vi "Binned Values.vi"(3 "Tolerance":dbl=1.0 format="%.2f", 4 "Precision (3)":string, 5 "String Array In":string[](array[string])) -> (2 "String Array Out":string[](array[string]))   [LabVIEW 2022 SP3]
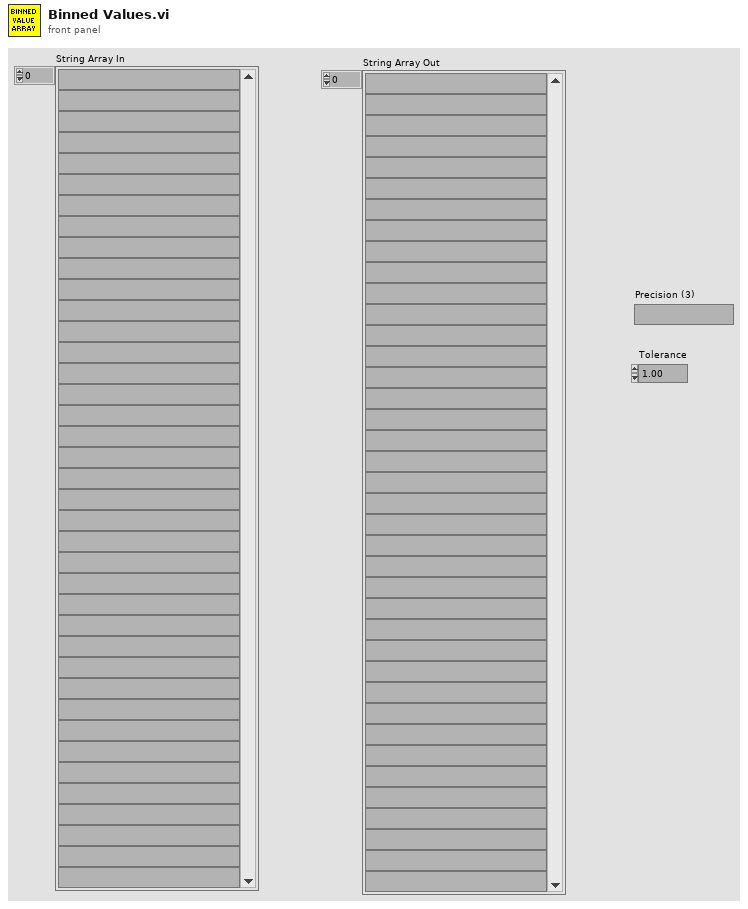
[diagram p1: front panel]
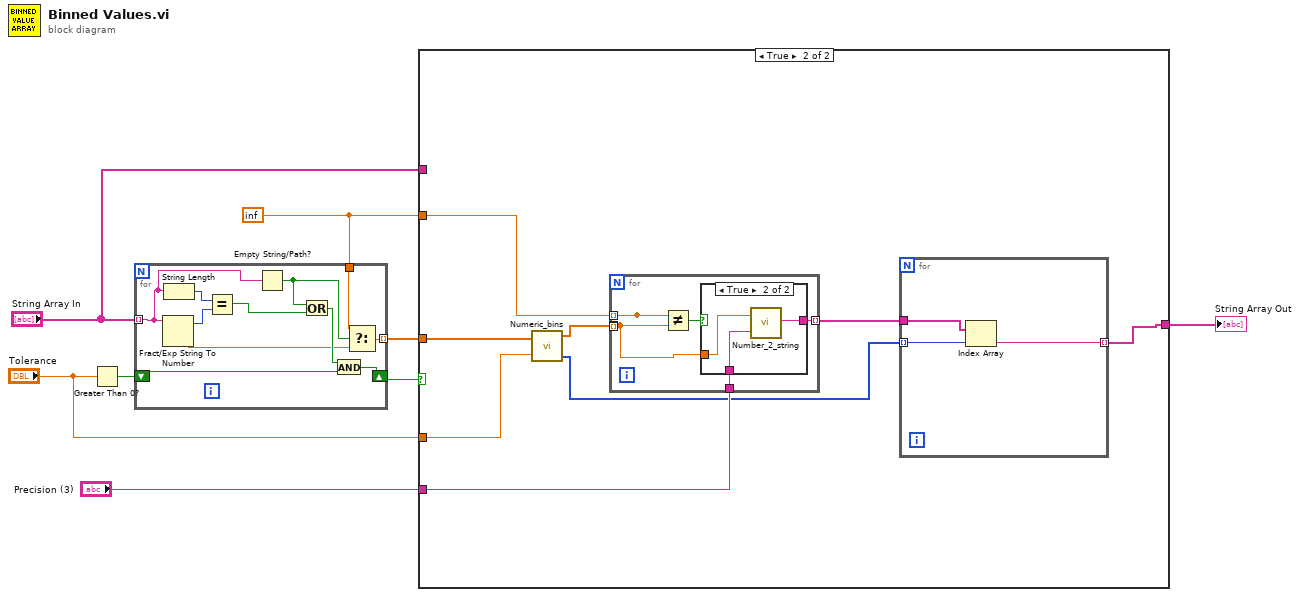
[diagram p0: block diagram]
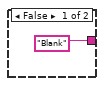
[diagram p3: hidden frame]
diagram:
  w2 = inf
  n1 = Greater Than 0?(x="Tolerance") -> (x > 0?=w8:bool)
  n2 = for {
    tunnel: "String Array In" -> [w10] mode=indexing
    shift-right: [w17] -> w7
    shift-left: w8 -> [w18]
    tunnel: [w14] -> w4 mode=indexing
    tunnel: w2 -> [w15]
    n3 = Fract/Exp String To Number(string=w10) -> (offset past number=w12:i32, number=w13:dbl)  [unwired: 3 out]
    n4 = String Length(string=w10) -> (length=w11:i32)
    n5 = Equal?(x=w11, y=w12) -> (x = y?=w9:bool)
    n6 = Empty String/Path?(string/path=w10) -> (empty?=w16:bool)
    n7 = Or(x=w16, y=w9) -> (x .or. y?=w19:bool)
    n8 = And(x=w19, y=w18) -> (x .and. y?=w17:bool)
    n9 = Select(t=w15, s=w16, f=w13) -> (s? t:f=w14:dbl)
  }
  n10 = case shown="True" w7 {
    tunnel: [w20 w21] -> w6
    tunnel: "String Array In" -> [w20 _]
    tunnel: w4 -> [_ w28]
    tunnel: "Tolerance" -> [_ w27]
    tunnel: w2 -> [_ w26]
    tunnel: "Precision (3)" -> [_ w24]
    frame False {
    }
    frame True {
      n11 = call "Numeric_bins.vi"("Values"=w28, "Tolerance"=w27) -> ("Bin Centres"=w25:dbl[], "Bin Index"=w22:i32[])  [unwired: 1 out]
      n12 = for {
        tunnel: w25 -> [w32] mode=indexing
        tunnel: w26 -> [w34]
        tunnel: [w35] -> w23 mode=indexing
        tunnel: [w32] -> _ mode=indexing
        tunnel: [w34] -> _ mode=indexing
        tunnel: w24 -> [w33]
        n13 = Not Equal?(x=w34, y=w32) -> (x != y?=w36:bool)
        n14 = case shown="True" w36 {
          tunnel: ["Blank" ("f") w40] -> w35
          tunnel: w32 -> [_ w39]
          tunnel: w33 -> [_ w38]
          frame False {
          }
          frame True {
            n15 = call "Number_2_string.vi"("precision"=w38, "number"=w39) -> ("String"=w40:string)
          }
        }
      }
      n16 = for {
        tunnel: w23 -> [w31]
        tunnel: w22 -> [w30] mode=indexing
        tunnel: [w29] -> w21 mode=indexing
        n17 = Index Array(array=w31, index=w30) -> (element=w29:string)
      }
    }
  }
  "String Array Out" <- w6
